vi "GenCM-List Connected Signals (Int32).vi"(0 "Path":path, 11 "error in (no error)":errorcluster) -> (4 "Analog Outputs":i32[](array[numeric]), 6 "Analog Inputs":i32[](array[numeric]), 8 "Digital Outputs":i32[](array[numeric]), 10 "Digital Inputs":i32[](array[numeric]), 15 "error out":errorcluster)   [LabVIEW 2015]
uses:
  <vilib>/Utility/config.llb/Read Key (I32).vi
  <vilib>/Utility/config.llb/NI_LVConfig.lvlib
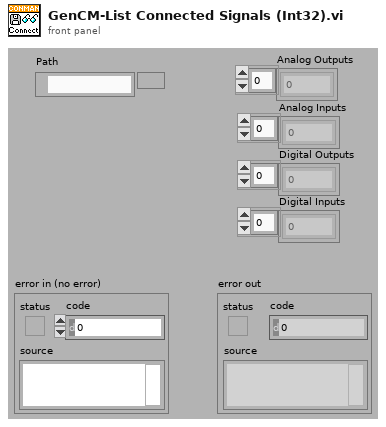
[diagram p1: front panel]
types:
  T1 = typedef "NI_LVConfig.lvlib/Config Data RefNum.ctl" = refnum<k1>
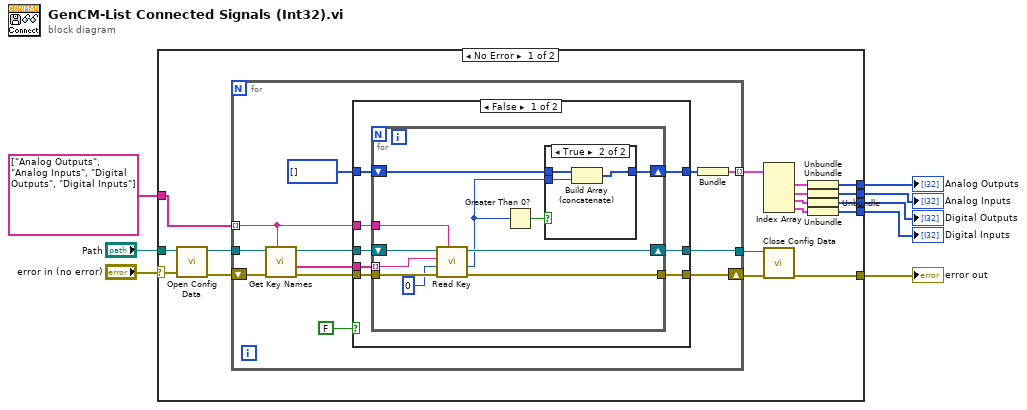
[diagram p0: block diagram]
diagram:
  n1 = case shown="No Error" "error in (no error)" {
    selector: "error in (no error)" -> [w25 w64]
    tunnel: [w24 w64] -> w7
    tunnel: "Path" -> [w23 _]
    tunnel: string[] ["Analog Outputs", "Analog Inputs", "Digital Outputs", "Digital Inputs"] -> [w22 _]
    tunnel: [w12 _] -> w4
    tunnel: [w11 _] -> w3
    tunnel: [w10 _] -> w2
    tunnel: [w9 _] -> w1
    frame No Error {
      n2 = call <vilib>:"Open Config Data.vi"("error in (no error)"=w25, "configuration file path"=w23) -> ("error out"=w18:errorcluster, "refnum"=w19:T1)  [unwired: 7 in, 1 out]
      n3 = for {
        tunnel: w19 -> [w33]
        tunnel: [w37] -> w21
        tunnel: w22 -> [w29] mode=indexing
        tunnel: [w26] -> w17 mode=indexing
        shift-right: [w36] -> w20
        shift-left: w18 -> [w32]
        n4 = call <vilib>:"Get Key Names.vi"("section"=w29, "error in (no error)"=w32, "refnum"=w33) -> ("error out"=w30:errorcluster, "key names"=w28:string[], "refnum out"=w31:T1)  [unwired: 5 in, 1 out]
        n5 = case shown="False" FALSE {
          tunnel: w31 -> [w45 w62]
          tunnel: i32[] [] -> [w44 w63]
          tunnel: [w43 w63] -> w35
          tunnel: [w42 w62] -> w37
          tunnel: w28 -> [w41 _]
          tunnel: w30 -> [w40 w61]
          tunnel: [w39 w61] -> w36
          tunnel: w29 -> [w38 _]
          frame False {
            n6 = for {
              tunnel: w41 -> [w48] mode=indexing
              shift-right: [w52] -> w43
              shift-left: w44 -> [w53]
              tunnel: w40 -> [w56]
              tunnel: [w50] -> w39
              tunnel: w38 -> [w47]
              shift-right: [w51] -> w42
              shift-left: w45 -> [w55]
              n7 = call-poly <vilib>:"Read Key.vi"("section"=w47, "error in (no error)"=w56, "default value"=0, "key"=w48, "refnum"=w55) -> ("error out"=w50:errorcluster, "value"=w46:i32, "refnum out"=w51:T1)  [unwired: 3 in, 1 out]
              n8 = Greater Than 0?(x=w46) -> (x > 0?=w49:bool)
              n9 = case shown="True" w49 {
                tunnel: w53 -> [w57 w60]
                tunnel: [w57 w59] -> w52
                tunnel: w46 -> [_ w58]
                frame False {
                }
                frame True {
                  n10 = Build Array (concatenate)(w60, w58) -> (w59:i32[])
                }
              }
            }
          }
          frame True {
          }
        }
        n11 = Bundle(w35) -> (w26:cluster{i32[]})  [unwired: 1 in]
      }
      n12 = Index Array(array=w17) -> (element #1=w16:cluster{i32[]}, element #2=w15:cluster{i32[]}, element #3=w14:cluster{i32[]}, element #4=w13:cluster{i32[]})  [unwired: 4 in]
      n13 = call <vilib>:"Close Config Data.vi"("error in (no error)"=w20, "refnum"=w21) -> ("error out"=w24:errorcluster)  [unwired: 8 in, 1 out]
      n14 = Unbundle(w16) -> (w12:i32[])
      n15 = Unbundle(w15) -> (w10:i32[])
      n16 = Unbundle(w14) -> (w11:i32[])
      n17 = Unbundle(w13) -> (w9:i32[])
    }
    frame Error {
    }
  }
  "error out" <- w7
  "Analog Outputs" <- w4
  "Analog Inputs" <- w2
  "Digital Outputs" <- w3
  "Digital Inputs" <- w1
